vi "Get Class Name.vi"(3 "lvclass":refnum<class>) -> (4 "Full Name":string, 5 "Child Name":string)   [LabVIEW 2025]
panel:
  out "class name":string
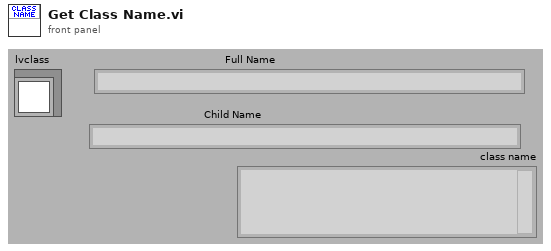
[diagram p1: front panel]
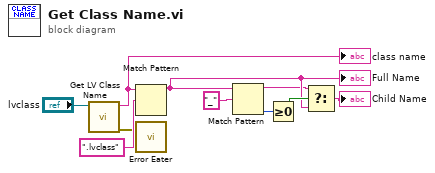
[diagram p0: block diagram]
diagram:
  n1 = call <vilib>:"Get LV Class Name.vi"("object"="lvclass") -> ("error out"=w6:errorcluster, "class name"=w7:string)  [unwired: 9 in]
  "class name" <- w7
  n2 = Match Pattern(string=w7, regular expression=".lvclass") -> (before substring=w2:string)  [unwired: 1 in, 3 out]
  "Full Name" <- w2
  n3 = call "Error Eater.vi"("error in (no error)"=w6) -> ()  [unwired: 2 in]
  n4 = Match Pattern(string=w2, regular expression="_") -> (before substring=w1:string, offset past match=w4:i32)  [unwired: 1 in, 2 out]
  n5 = Greater Or Equal To 0?(x=w4) -> (x >= 0?=w3:bool)
  n6 = Select(t=w1, s=w3, f=w2) -> (s? t:f=→"Child Name":string)
